vi "Get if acquring.vi"(8 "error in (no error)":errorcluster, 11 "DAQCascade512II in":refnum<class "DAQCascade512II.lvclass">) -> (0 "error out":errorcluster, 3 "DAQCascade512II out":refnum<class "DAQCascade512II.lvclass">)   [LabVIEW 2012, in "DAQCascade512II.lvclass"]
doc: "Returns the settings path."
uses:
  DAQCascade512II.lvclass
  DAQCascade512II.lvclass/DAQCascade512II.ctl
panel:
  out "Acquire mode?":bool
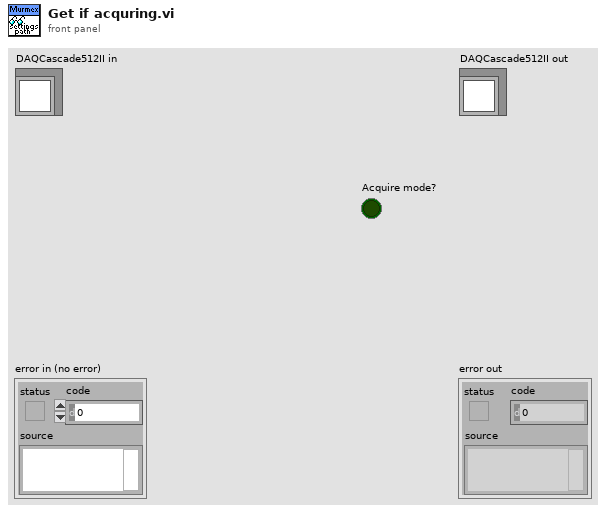
[diagram p1: front panel]
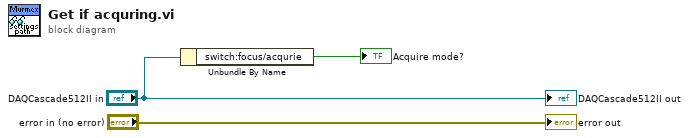
[diagram p0: block diagram]
diagram:
  n1 = Unbundle By Name("DAQCascade512II in") -> ("switch:focus/acqurie"=→"Acquire mode?":bool)
  "error out" <- "error in (no error)"
  "DAQCascade512II out" <- "DAQCascade512II in"
